vi "test Diff Configuration (No Change).vi"(8 "error in":errorcluster, 11 "TestCase in":refnum<class "Refresh.lvclass">) -> (0 "error out":errorcluster, 3 "TestCase out":refnum<class "Refresh.lvclass">)   [LabVIEW 2020, in "Refresh.lvclass"]
uses:
  Refresh.lvclass
  <vilib>/addons/_JKI Toolkits/VI Tester/TestCase.llb/TestCase.lvclass
  System Explorer/Implementation/System Explorer/Refresh/Refresh.lvlib
  Shared/Parameter Definition.ctl
  Shared/Address.ctl
  Shared/Terminal Endpoint.ctl
  Shared/Message Type.ctl
  Shared/Message Definition.ctl
  Shared/1553 Channel.ctl
  System Explorer/Implementation/System Explorer/Refresh/Change Type.ctl
  C:/Program Files (x86)/National Instruments/LabVIEW 2020/vi.lib/addons/_JKI Toolkits/VI Tester/TestCase.llb/TestCase.lvclass
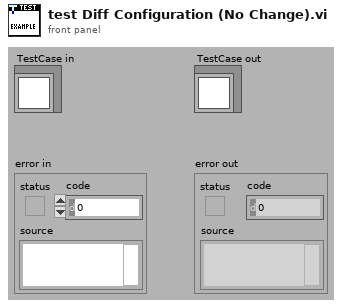
[diagram p1: front panel]
types:
  T1 = typedef "1553 Channel.ctl" = cluster{"HW channel":u16, "bus controller address":i16, "terminal addresses":T2[], "terminal names":string[], "acyclic frame names":string[], "messages":T3[]}
  T2 = typedef "Address.ctl" = u16
  T3 = typedef "Message Definition.ctl" = cluster{"name":string, "message type":T4, "endpoint Tx":T5, "endpoint Rx":T5, "create timestamp channel":bool, "mode code":u16, "number of words":u16, "parameters":cluster{"name":string, "default value":dbl, "unit":string, "parameter definition":T6}[]}
  T4 = typedef "Message Type.ctl" = string
  T5 = typedef "Terminal Endpoint.ctl" = cluster{"terminal address":T2, "subaddress":T2}
  T6 = typedef "Parameter Definition.ctl" = cluster{"start index":i32, "size (bits)":i32, "encoding":enum16{"BNR", "BCD", "Discrete"}, "signed":bool, "multiplier":dbl, "offset":dbl}
  T7 = typedef "Ballard MIL-STD-1553 System Explorer.lvlib/Implementation.lvlib/Refresh.lvlib/Change Type.ctl" = enum16{"No change", "Modify", "Add", "Remove"}
  T8 = typedef "Ballard MIL-STD-1553 System Explorer.lvlib/Implementation.lvlib/Refresh.lvlib/MCL Row.ctl" = cluster{"change type":T7, "item symbol":T9, "item names":string[]}
  T9 = typedef "Ballard MIL-STD-1553 System Explorer.lvlib/Implementation.lvlib/Refresh.lvlib/Symbols.ctl" = enum16{"Blank", "MIL-STD-1553", "Port", "Remote Terminal", "Subaddress", "Bus Controller", "Acyclic Frame", "Mode Code", "Message", "Parameter", "Item"}
  T10 = cluster{"name":string, "default value":dbl, "unit":string, "parameter definition":T6}[]
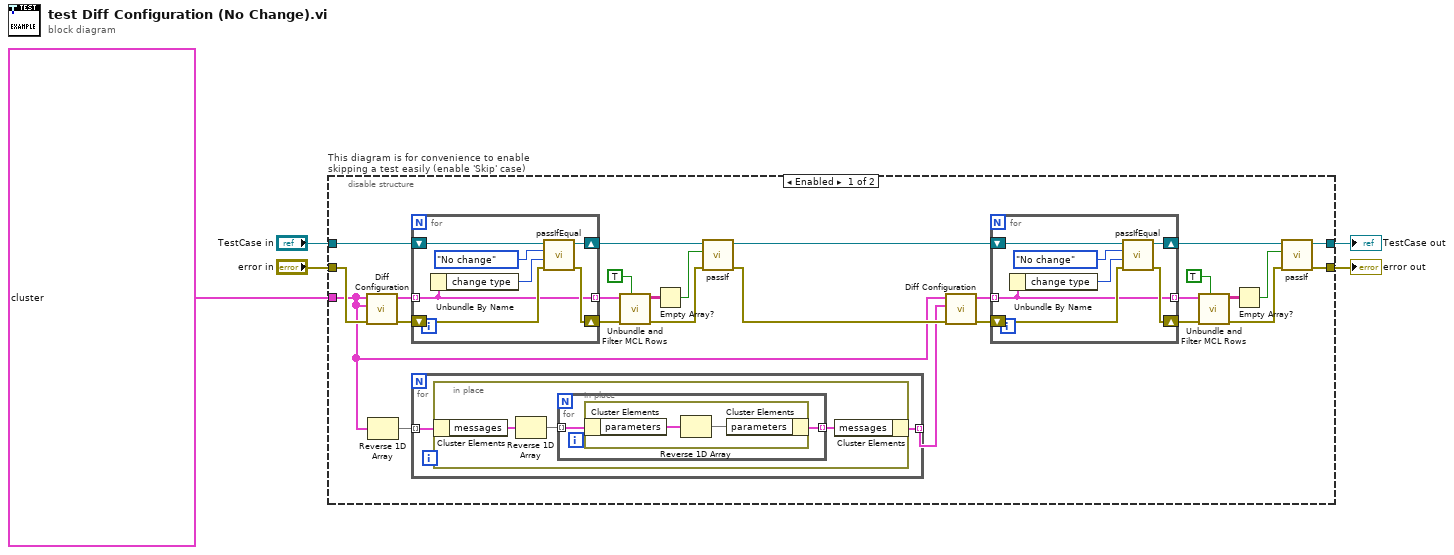
[diagram p0: block diagram]
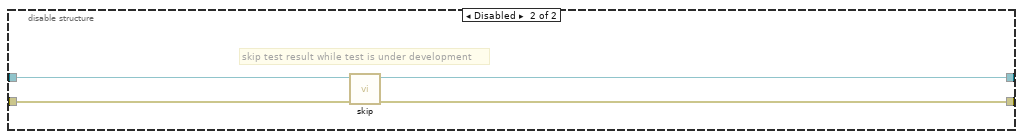
[diagram p2: hidden frame]
diagram:
  n1 = disable-structure "This diagram is for convenience to enable skipping a test easily (enable 'Skip' case)" shown="Enabled" {
    disable-tunnel: "TestCase in" -> [w31 w59]
    disable-tunnel: [w6 w57] -> w2
    disable-tunnel: [w7 w58] -> w4
    disable-tunnel: "error in" -> [w32 w56]
    disable-tunnel: T1[] [{"HW channel"=0, "bus controller address"=0, "terminal addresses"=[0, 1, 2], "terminal names"=[], "acyclic frame names"=[], "messages"=[{"name"="Message 001", "message type"="BC to RT", "endpoint Tx"={"terminal address"=1, "subaddress"=1}, "endpoint Rx"={"terminal address"=0, "subaddress"=0}, "create timestamp channel"=TRUE, "mode code"=0, "number of words"=3, "parameters"=[{"name"="Word0", "default value"=1.0, "unit"="eu", "parameter definition"={"start index"=0, "size (bits)"=16, "encoding"=enum."BNR", "signed"=FALSE, "multiplier"=1.0, "offset"=0.0}}, {"name"="Word1", "default value"=1.0, "unit"="eu", "parameter definition"={"start index"=16, "size (bits)"=16, "encoding"=enum."BNR", "signed"=TRUE, "multiplier"=1.0, "offset"=0.0}}, {"name"="Word2", "default value"=1.0, "unit"="eu", "parameter definition"={"start index"=32, "size (bits)"=16, "encoding"=enum."BNR", "signed"=TRUE, "multiplier"=1.0, "offset"=0.0}}]}]}, {"HW channel"=1, "bus controller address"=0, "terminal addresses"=[10, 11], "terminal names"=[], "acyclic frame names"=[], "messages"=[{"name"="RT 10.10 to RT 11.11", "message type"="RT to RT", "endpoint Tx"={"terminal address"=11, "subaddress"=1}, "endpoint Rx"={"terminal address"=10, "subaddress"=10}, "create timestamp channel"=FALSE, "mode code"=0, "number of words"=2, "parameters"=[{"name"="P0", "default value"=1.0, "unit"="freedom units", "parameter definition"={"start index"=0, "size (bits)"=32, "encoding"=enum."BNR", "signed"=TRUE, "multiplier"=1.0, "offset"=0.0}}]}]}] ("configuration old") -> [w9 _]
    frame Enabled {
      n2 = call "Diff Configuration.vi"("error in"=w32, "configuration new"=w9, "configuration old"=w9) -> ("error out"=w26:errorcluster, "configuration diff"=w25:T8[])  [unwired: 7 in]
      n3 = Reverse 1D Array(array=w9) -> (reversed array=w21:T1[])
      n4 = for {
        shift-right: [w54] -> w27
        shift-left: w31 -> [w55]
        shift-right: [w50] -> w23
        shift-left: w26 -> [w51]
        tunnel: w25 -> [w49] mode=indexing
        tunnel: [w49] -> w24 mode=indexing
        n5 = Unbundle By Name(w49) -> ("change type"=w52:T7)
        n6 = call-dynamic "passIfEqual.vi"("error in (no error)"=w51, "y"=w52, "x"=Change_Type."No change" ("change type"), "TestCase in"=w55) -> ("error out"=w50:errorcluster, "TestCase out"=w54:refnum<class "Refresh.lvclass">)  [unwired: 6 in]
      }
      n7 = for {
        tunnel: w21 -> [w41] mode=indexing
        tunnel: [w40] -> w8 mode=indexing
        n8 = in-place {
          n9 = in-place-cluster #1(w41) -> ("messages"=w43:T3[])
          n10 = Reverse 1D Array(array=w43) -> (reversed array=w44:T3[])
          n11 = for {
            tunnel: w44 -> [w46] mode=indexing
            tunnel: [w45] -> w42 mode=indexing
            n12 = in-place {
              n13 = in-place-cluster #2(w46) -> ("parameters"=w48:T10)
              n14 = Reverse 1D Array(array=w48) -> (reversed array=w47:T10)
              n15 = in-place-cluster #2("parameters"=w47) -> (w45:T3)
            }
          }
          n16 = in-place-cluster #1("messages"=w42) -> (w40:T1)
        }
      }
      n17 = call "Unbundle and Filter MCL Rows.vi"("filter changed items"=TRUE, "error in"=w23, "refresh items"=w24) -> ("error out"=w22:errorcluster, "item names"=w29:string[][])  [unwired: 5 in, 2 out]
      n18 = Empty Array?(array=w29) -> (empty?=w28:bool)
      n19 = call-dynamic "passIf.vi"("error in (no error)"=w22, "pass"=w28, "TestCase in"=w27) -> ("error out"=w10:errorcluster, "TestCase out"=w11:refnum<class "Refresh.lvclass">)  [unwired: 7 in]
      n20 = call "Diff Configuration.vi"("error in"=w10, "configuration new"=w8, "configuration old"=w9) -> ("error out"=w16:errorcluster, "configuration diff"=w17:T8[])  [unwired: 7 in]
      n21 = for {
        shift-right: [w38] -> w15
        shift-left: w11 -> [w39]
        shift-right: [w34] -> w19
        shift-left: w16 -> [w35]
        tunnel: w17 -> [w33] mode=indexing
        tunnel: [w33] -> w18 mode=indexing
        n22 = Unbundle By Name(w33) -> ("change type"=w36:T7)
        n23 = call-dynamic "passIfEqual.vi"("error in (no error)"=w35, "y"=w36, "x"=Change_Type."No change" ("change type"), "TestCase in"=w39) -> ("error out"=w34:errorcluster, "TestCase out"=w38:refnum<class "Refresh.lvclass">)  [unwired: 6 in]
      }
      n24 = call "Unbundle and Filter MCL Rows.vi"("filter changed items"=TRUE, "error in"=w19, "refresh items"=w18) -> ("error out"=w20:errorcluster, "item names"=w13:string[][])  [unwired: 5 in, 2 out]
      n25 = Empty Array?(array=w13) -> (empty?=w14:bool)
      n26 = call-dynamic "passIf.vi"("error in (no error)"=w20, "pass"=w14, "TestCase in"=w15) -> ("error out"=w7:errorcluster, "TestCase out"=w6:refnum<class "Refresh.lvclass">)  [unwired: 7 in]
    }
    frame Disabled {
      # "skip test result while test is under development"
      n27 = call <vilib>:"skip.vi"("error in (no error)"=w56, "TestCase in"=w59) -> ("error out"=w58:errorcluster, "TestCase out"=w57:refnum<class "Refresh.lvclass">)  [unwired: 8 in]
    }
  }
  "error out" <- w4
  "TestCase out" <- w2
